vi "produceTimingTicks.vi"(8 "error in (no error)":errorcluster, 10 "Channel":refnum<class "Channel.lvclass">, 11 "RfRamp in":refnum<class "RfRamp.lvclass">) -> (0 "error out":errorcluster, 2 "timingTick":refnum<class "ScriptEventList.lvclass">, 3 "RfRamp out":refnum<class "RfRamp.lvclass">)   [LabVIEW 2011, in "Tools.lvlib" / "Scripting.lvlib" / "RfRamp.lvclass"]
uses:
  RfRamp.lvclass
  DatabaseHelpers/Database Objects/Channel/Channel.lvclass
  ScriptEventList/ScriptEventList.lvclass
  ScriptEvent.lvclass
  RfRamp.lvclass/RfRamp.ctl
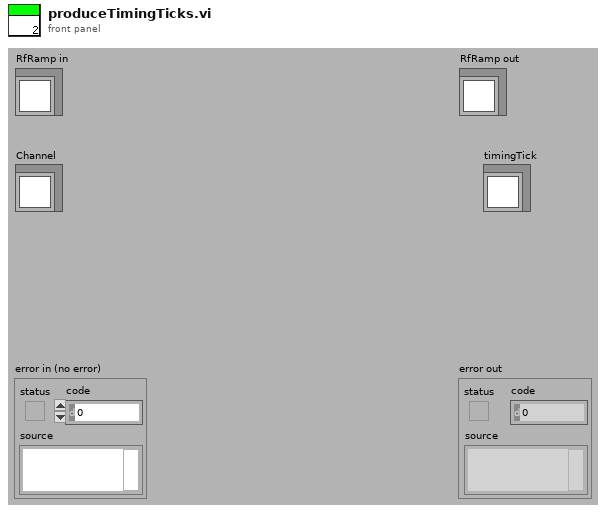
[diagram p1: front panel]
types:
  T1 = enum16{"changeValue", "pulse", "clock", "rampUp", "rampDown", "singleTone", "singleToneRamp", "playFile", "rf", "rfRamp"}
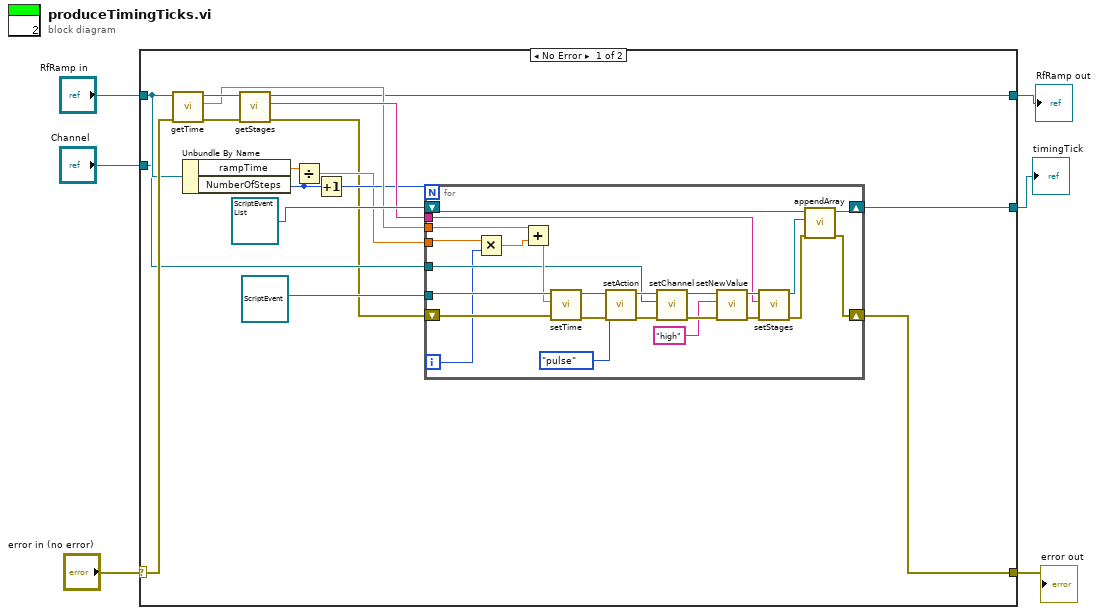
[diagram p0: block diagram]
diagram:
  n1 = case shown="No Error" "error in (no error)" {
    selector: "error in (no error)" -> [w23 w48]
    tunnel: "RfRamp in" -> [w22 w49]
    tunnel: [w10 w49] -> w4
    tunnel: "Channel" -> [w17 _]
    tunnel: [w8 w48] -> w2
    tunnel: [w11 _] -> w1
    frame No Error {
      n2 = call "getTime.vi"("error in (no error)"=w23, "ScriptEvent.lvclass in"=w22) -> ("error out"=w19:errorcluster, "time"=w15:dbl, "ScriptEvent.lvclass out"=w20:refnum<class "RfRamp.lvclass">)  [unwired: 7 in]
      n3 = Unbundle By Name(w22) -> ("rampTime"=w14:dbl, "NumberOfSteps"=w7:i32)
      n4 = call "getStages.vi"("error in (no error)"=w19, "ScriptEvent.lvclass in"=w20) -> ("error out"=w9:errorcluster, "Stage"=w18:string, "ScriptEvent.lvclass out"=w10:refnum<class "RfRamp.lvclass">)  [unwired: 7 in]
      n5 = Divide(x=w14, y=w7) -> (x/y=w12:dbl)
      n6 = Increment(x=w7) -> (x+1=w13:i32)
      n7 = for {
        N: w13 -> [_]
        tunnel: w12 -> [w46]
        tunnel: w15 -> [w47]
        tunnel: refnum<class "ScriptEvent.lvclass"> refnum ("Tools.lvlib:Scripting.lvlib:ScriptEvent.lvclass") -> [w44]
        tunnel: w17 -> [w37]
        shift-right: [w30] -> w8
        shift-left: w9 -> [w42]
        shift-right: [w32] -> w11
        shift-left: refnum<class "ScriptEventList.lvclass"> refnum ("Tools.lvlib:Scripting.lvlib:ScriptEventList.lvclass") -> [w31]
        tunnel: w18 -> [w25]
        i -> [w33]
        n8 = Multiply(x=w46, y=w33) -> (x*y=w45:dbl)
        n9 = Add(x=w47, y=w45) -> (x+y=w43:dbl)
        n10 = call "setTime.vi"("error in (no error)"=w42, "time"=w43, "ScriptEvent.lvclass in"=w44) -> ("error out"=w40:errorcluster, "ScriptEvent.lvclass out"=w41:refnum<class "ScriptEvent.lvclass">)  [unwired: 7 in]
        n11 = call "setAction.vi"("error in (no error)"=w40, "action"=T1."pulse", "ScriptEvent.lvclass in"=w41) -> ("error out"=w38:errorcluster, "ScriptEvent.lvclass out"=w39:refnum<class "ScriptEvent.lvclass">)  [unwired: 7 in]
        n12 = call-dynamic "setChannel.vi"("error in (no error)"=w38, "Channel.lvclass"=w37, "ScriptEvent.lvclass in"=w39) -> ("error out"=w35:errorcluster, "ScriptEvent.lvclass out"=w36:refnum<class "ScriptEvent.lvclass">)  [unwired: 7 in]
        n13 = call "setNewValue.vi"("error in (no error)"=w35, "newValue"="high", "ScriptEvent.lvclass in"=w36) -> ("error out"=w28:errorcluster, "ScriptEvent.lvclass out"=w29:refnum<class "ScriptEvent.lvclass">)  [unwired: 7 in]
        n14 = call-dynamic "setStages.vi"("error in (no error)"=w28, "Stage"=w25, "ScriptEvent.lvclass in"=w29) -> ("error out"=w27:errorcluster, "ScriptEvent.lvclass out"=w26:refnum<class "ScriptEvent.lvclass">)  [unwired: 7 in]
        n15 = call "appendArray.vi"("error in (no error)"=w27, "ScriptEvent"=w26, "ScriptEventList in"=w31) -> ("error out"=w30:errorcluster, "ScriptEventList out"=w32:refnum<class "ScriptEventList.lvclass">)  [unwired: 6 in, 1 out]
      }
    }
    frame Error {
    }
  }
  "error out" <- w2
  "RfRamp out" <- w4
  "timingTick" <- w1
